vi "NIDIO Test Harness.vi"() -> ()   [LabVIEW 2015, in "NIDIO.lvclass"]
uses:
  NIDIO.lvclass
  Galvo/NI Galvo/NI Galvo.lvclass
  Laser/Axsun/1310/Axsun_1310_SS.lvclass
  Galvo/Scanning Cluster.ctl
  Galvo/Galvo.lvclass
  DAQ/Trigger Source.ctl
  DAQ/DAQ Class.lvclass
  DAQ/Trigger Slope.ctl
  Type Defs/OCT DAQ Channel Data Type.ctl
  DAQ/Clock Control.ctl
  DAQ/DAQ Parameters.ctl
panel:
  out "Waveform Graph":waveform(i32)(graph)
  in  "Stop A-Scan":u32
  in  "Start A-Scan":u32
  in  "Scan Button":bool caption="Blank Button"
  in  "Quit Button":bool
  in  "NIDIO in":refnum<class "NIDIO.lvclass">
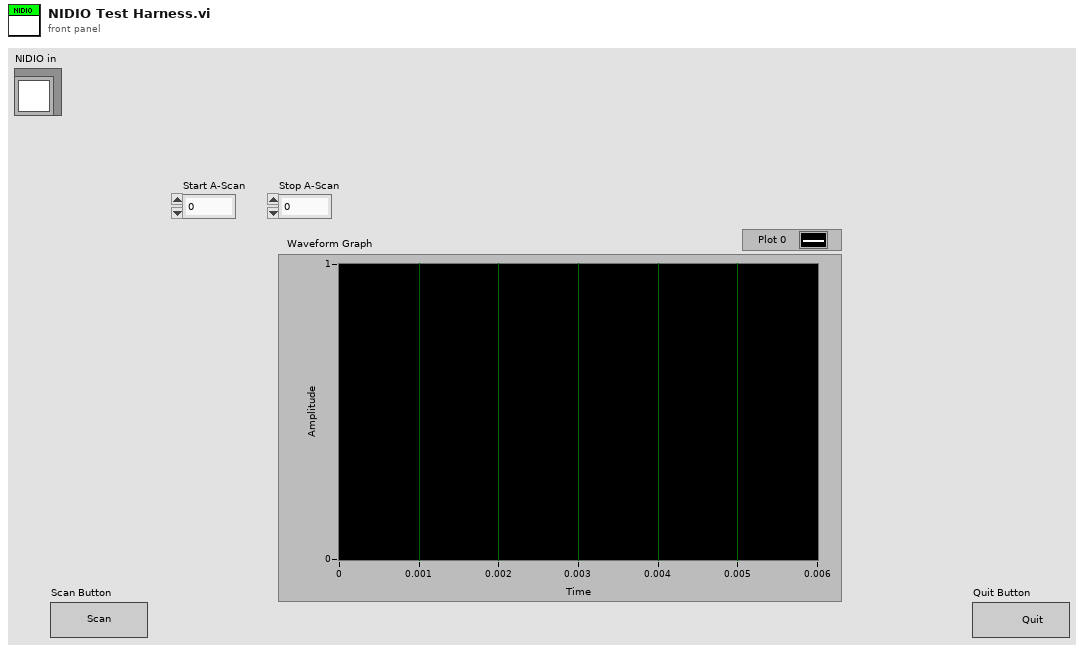
[diagram p1: front panel]
types:
  T1 = typedef "DAQ Class.lvclass/DAQ Parameters.ctl" = cluster{"Points Per A-Scan":u32, "A-Scans Per B-Scan":u32, "Number of B-Scans":u32, "B-Scans Per Transfer":u32, "Trigger Voltage":sgl, "Trigger Source":T2, "Trigger Slope":T3, "Channel":T4, "Clock":T5, "Bits per Sample":dbl, "Range":dbl, "Start Trim":u32, "Stop Trim":u32}
  T2 = typedef "DAQ Class.lvclass/Trigger Source.ctl" = enum16{"External", "Channel A", "Channel B"}
  T3 = typedef "DAQ Class.lvclass/Trigger Slope.ctl" = enum16{"Rising", "Falling"}
  T4 = typedef "OCT DAQ Channel Data Type.ctl" = enum16{"Channel 1", "Channel 2", "Channel 1 and 2"}
  T5 = typedef "DAQ Class.lvclass/Clock Control.ctl" = enum16{"Internal Clock", "External Clock"}
  T6 = typedef "Galvo.lvclass/Scanning Cluster.ctl" = cluster{"Fast Axis Offset":sgl, "Slow Axis Offset":sgl, "Slow Axis Amp":sgl, "Fast Axis Amp":sgl, "Scan Pattern":enum16{"Raster", "Triangle Raster", "Sinusoid Raster"}}
  T7 = typedef "Galvo.lvclass/Fast Axis Parameters.ctl" = cluster{"Fast Axis Voltage":dbl, "Laser Sweep Frequency":dbl, "A-Scans in Fast Axis":dbl}
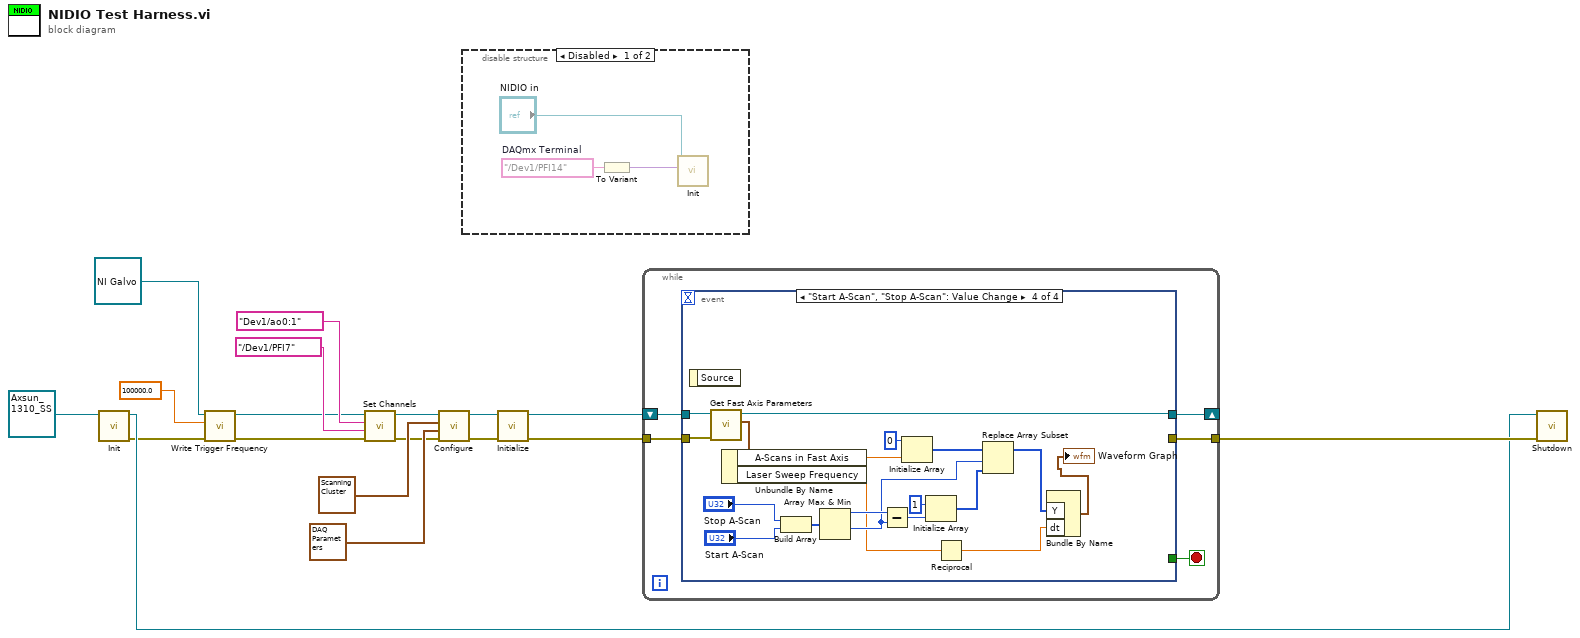
[diagram p0: block diagram]
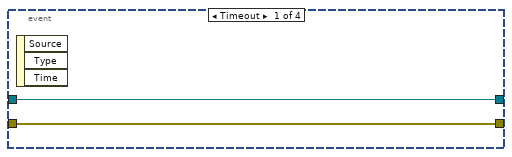
[diagram p2: hidden frame]
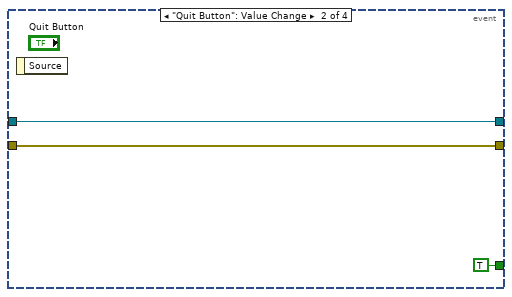
[diagram p3: hidden frame]
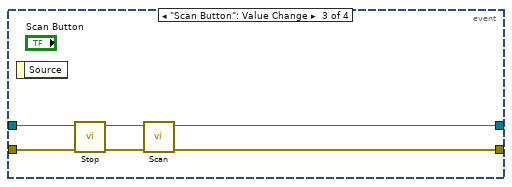
[diagram p4: hidden frame]
diagram:
  n1 = call-dynamic "Init.vi"("Axsun_1310_SS in"=refnum<class "Axsun_1310_SS.lvclass"> refnum ("Axsun_1310_SS.lvclass")) -> ("error out"=w7:errorcluster, "Axsun_1310_SS out"=w14:refnum<class "Axsun_1310_SS.lvclass">)  [unwired: 9 in]
  n2 = call-dynamic "Write Trigger Frequency.vi"("error in (no error)"=w7, "Trigger Frequency"=100000.0, "Galvo in"=refnum<class "NI Galvo.lvclass"> refnum ("NI Galvo.lvclass")) -> ("error out"=w6:errorcluster, "Galvo out"=w4:refnum<class "NI Galvo.lvclass">)  [unwired: 7 in]
  n3 = call-dynamic "Set Channels.vi"("error in (no error)"=w6, "Trigger Source"=tag "/Dev1/PFI7", "Analog Output"=tag "Dev1/ao0:1", "NI Galvo in"=w4) -> ("error out"=w11:errorcluster, "NI Galvo out"=w10:refnum<class "NI Galvo.lvclass">)  [unwired: 6 in]
  n4 = call-dynamic "Configure.vi"("error in (no error)"=w11, "DAQ Parameters"=T1 {"Points Per A-Scan"=512, "A-Scans Per B-Scan"=512, "Number of B-Scans"=512, "B-Scans Per Transfer"=512, "Trigger Voltage"=0.0, "Trigger Source"=enum."External", "Trigger Slope"=enum."Rising", "Channel"=enum."Channel 1", "Clock"=enum."Internal Clock", "Bits per Sample"=0.0, "Range"=0.0, "Start Trim"=0, "Stop Trim"=0}, "Scanning Parameters"=T6 {"Fast Axis Offset"=-2.5, "Slow Axis Offset"=-2.5, "Slow Axis Amp"=5.0, "Fast Axis Amp"=5.0, "Scan Pattern"=enum."Raster"}, "NI Galvo in"=w10) -> ("error out"=w8:errorcluster, "NI Galvo out"=w9:refnum<class "NI Galvo.lvclass">)  [unwired: 6 in]
  n5 = disable-structure shown="Disabled" {
    frame Disabled {
      w21 = tag "/Dev1/PFI14"  # DAQmx Terminal
      n6 = To Variant(anything=w21) -> (Variant=w20:variant)
      n7 = call-dynamic "Init.vi"("DIO Configuration In"=w20, "NIDIO in"="NIDIO in") -> ()  [unwired: 8 in, 2 out]
    }
    frame Enabled {
    }
  }
  n8 = call-dynamic "Initialize.vi"("error in (no error)"=w8, "NI Galvo in"=w9) -> ("error out"=w1:errorcluster, "NI Galvo out"=w2:refnum<class "NI Galvo.lvclass">)  [unwired: 8 in]
  n9 = while {
    tunnel: w1 -> [w24]
    shift-right: [w22] -> _
    shift-left: w2 -> [w25]
    tunnel: [w23] -> w15
    stop <- w26 stop-if-true
    n10 = event shown="[3] \"Start A-Scan\", \"Stop A-Scan\": Value Change" {
      selector: _ -> [_ _ _ _]
      dyn-events: _ -> [_ _ _ _]
      timeout: _ -> [_ _ _ _]
      tunnel: [_ TRUE _ _] -> w26
      tunnel: w25 -> [w27 w29 w35 w55]
      tunnel: w24 -> [w28 w30 w34 w56]
      tunnel: [w28 w30 w37 _] -> w23
      tunnel: [w27 w29 w36 w42] -> w22
      event Timeout {
        n11 = event-data() -> ()  [unwired: 1 in, 3 out]
      }
      event "Quit Button": Value Change {
        n12 = event-data() -> ()  [unwired: 1 in, 1 out]
      }
      event "Scan Button": Value Change {
        n13 = event-data() -> ()  [unwired: 1 in, 1 out]
        n14 = call-dynamic "Stop.vi"("error in (no error)"=w34, "NI Galvo in"=w35) -> ("error out"=w32:errorcluster, "NI Galvo out"=w33:refnum<class "NI Galvo.lvclass">)  [unwired: 8 in]
        n15 = call-dynamic "Scan.vi"("error in (no error)"=w32, "NI Galvo in"=w33) -> ("error out"=w37:errorcluster, "NI Galvo out"=w36:refnum<class "NI Galvo.lvclass">)  [unwired: 8 in]
      }
      event "Start A-Scan", "Stop A-Scan": Value Change {
        n16 = event-data() -> ()  [unwired: 1 in, 1 out]
        n17 = call-dynamic "Get Fast Axis Parameters.vi"("error in (no error)"=w56, "Galvo in"=w55) -> ("Fast Axis Parameters"=w48:T7, "Galvo out"=w42:refnum<class "NI Galvo.lvclass">)  [unwired: 7 in, 1 out]
        n18 = Unbundle By Name(w48) -> ("A-Scans in Fast Axis"=w47:dbl, "Laser Sweep Frequency"=w41:dbl)
        n19 = Build Array("Stop A-Scan", "Start A-Scan") -> (w52:u32[])
        n20 = Array Max & Min(array=w52) -> (max value=w51:u32, min value=w44:u32)  [unwired: 2 out]
        n21 = Subtract(x=w51, y=w44) -> (x-y=w50:u32)
        n22 = Initialize Array(0 ("element"), w47) -> (w45:i32[])
        n23 = Initialize Array(1 ("element"), w50) -> (w43:i32[])
        n24 = Reciprocal(x=w41) -> (1/x=w40:dbl)
        n25 = Replace Array Subset(array=w45, new element=w43, index=w44) -> (w39:i32[])
        n26 = Bundle By Name("Y"=w39, "dt"=w40) -> (→"Waveform Graph":waveform(i32))  [unwired: 1 in]
      }
    }
  }
  n27 = call-dynamic "Shutdown.vi"("error in (no error)"=w15, "Axsun_1310_SS in"=w14) -> ()  [unwired: 8 in, 2 out]
